vi "String to Complex Number (CSG).vi"(2 "use system decimal point (T)":bool=TRUE, 3 "default (0 CDB)":csg, 4 "offset":i32, 5 "string":string) -> (0 "number":csg, 1 "offset past number":i32)   [LabVIEW 2018, in "Numeric Data Type.lvclass"]
doc: "<b> </b> <b> </b>\n©2013, Q Software Innovations, LLC.\n\nWritten in National Instruments LabVIEW™ 2013.\n\nAuthored by Quentin Alldredge\nQ@qsoftwareinnovations.com\nwww.qsoftwareinnovations.com\n\nAll rights reserved."
uses:
  Numeric Data Type.lvclass
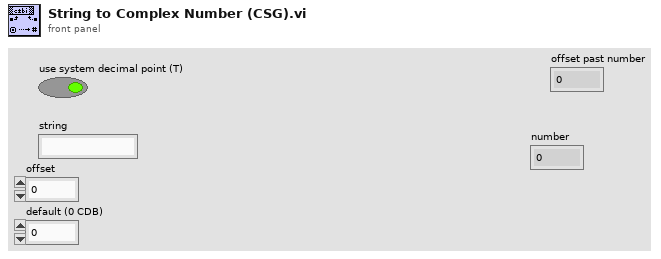
[diagram p1: front panel]
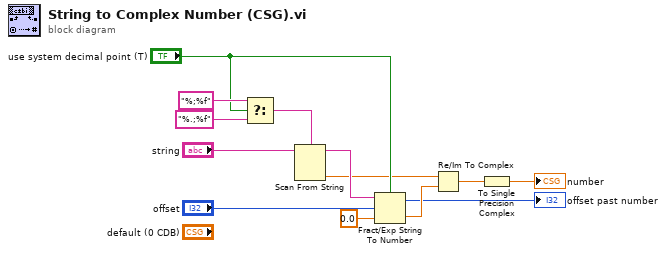
[diagram p0: block diagram]
diagram:
  n1 = Select(t="%;%f", s="use system decimal point (T)", f="%.;%f") -> (s? t:f=w11:string)
  n2 = Scan From String(format string=w11, input string="string") -> (remaining string=w9:string, output 1=w7:dbl)  [unwired: 3 in, 2 out]
  n3 = Fract/Exp String To Number(use system decimal point (T)="use system decimal point (T)", string=w9, offset="offset", default (0 dbl)=0.0 ("default (0 DBL)")) -> (offset past number=→"offset past number":i32, number=w6:dbl)
  n4 = Re/Im To Complex(1:w6, 2:w7) -> (0:w4:cdb)
  n5 = To Single Precision Complex(1:w4) -> (0:→"number":csg)
